vi "PICRv1.1.vi"() -> ()   [LabVIEW 2013]
uses:
  <vilib>/userdefined/High Color/IMAQdx.ctl
  <vilib>/LabVIEW Interface for Arduino/Type Defs/Board Type.ctl
  <vilib>/LabVIEW Interface for Arduino/Type Defs/Connection Type.ctl
  <vilib>/vision/driver/NI_Vision_Acquisition_Software.lvlib
  <vilib>/LabVIEW Interface for Arduino/LabVIEW Interface for Arduino.lvlib
panel:
  in  "Enum":enum16{"", "Forward", "Back"}(ring)
  in  "VISA resource":refnum<visa-resource-name>
  in  "Play 2":bool
  in  "Back 2":bool
  in  "Forward 2":bool
  in  "Play":bool
  in  "Back":bool
  in  "Forward":bool
  in  "Speed Control - Brush":dbl(knob) scale=0.0..100.0
  out "Speed - Brush":dbl(knob) scale=0.0..100.0
  in  "Speed Control - Motors":dbl(knob) scale=0.0..100.0
  out "Speed - Motors":dbl(knob) scale=0.0..100.0
  in  "Stop":bool
  out "Image":T1(plugin-control)
  in  "Session In":T2
  # "Motion"
  # "IMU"
  # "Camera"
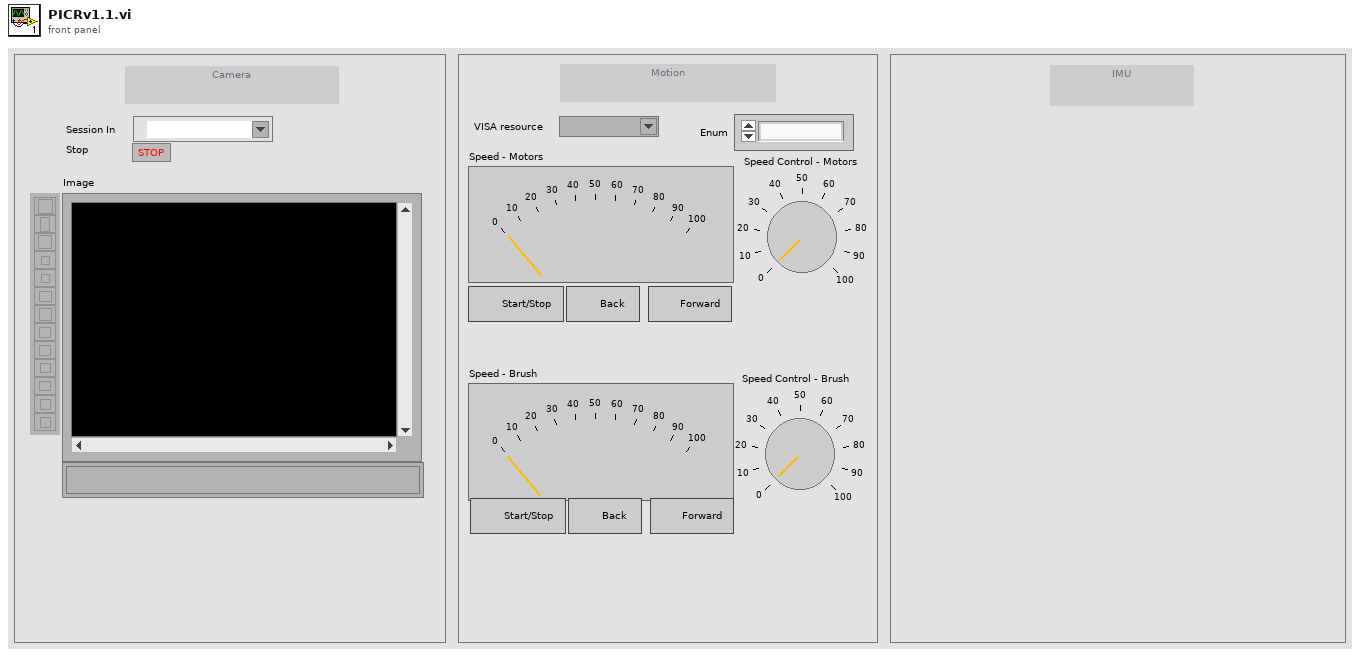
[diagram p1: front panel]
types:
  T1 = typedef "IMAQ Image.ctl" = refnum<image>
  T2 = typedef "IMAQdx.ctl" = refnum<k21>
  T3 = typedef "LabVIEW Interface for Arduino.lvlib/Connection Type.ctl" = enum8{"USB / Serial", "XBEE", "BlueSmirf (Bluetooth)"}
  T4 = typedef "LabVIEW Interface for Arduino.lvlib/Board Type.ctl" = enum16{"Uno", "Dimuelanove w/Atmega 328", "Mega 2560"}
  T5 = typedef "Image Type" = u32
  T6 = typedef "LabVIEW Interface for Arduino.lvlib/Arduino Resource.ctl" = cluster{"VISA resource":refnum<visa-resource-name>, "Board Type":T4, "Connection Type":enum8{"USB / Serial"}, "Bytes Per Packet (15)":u8}
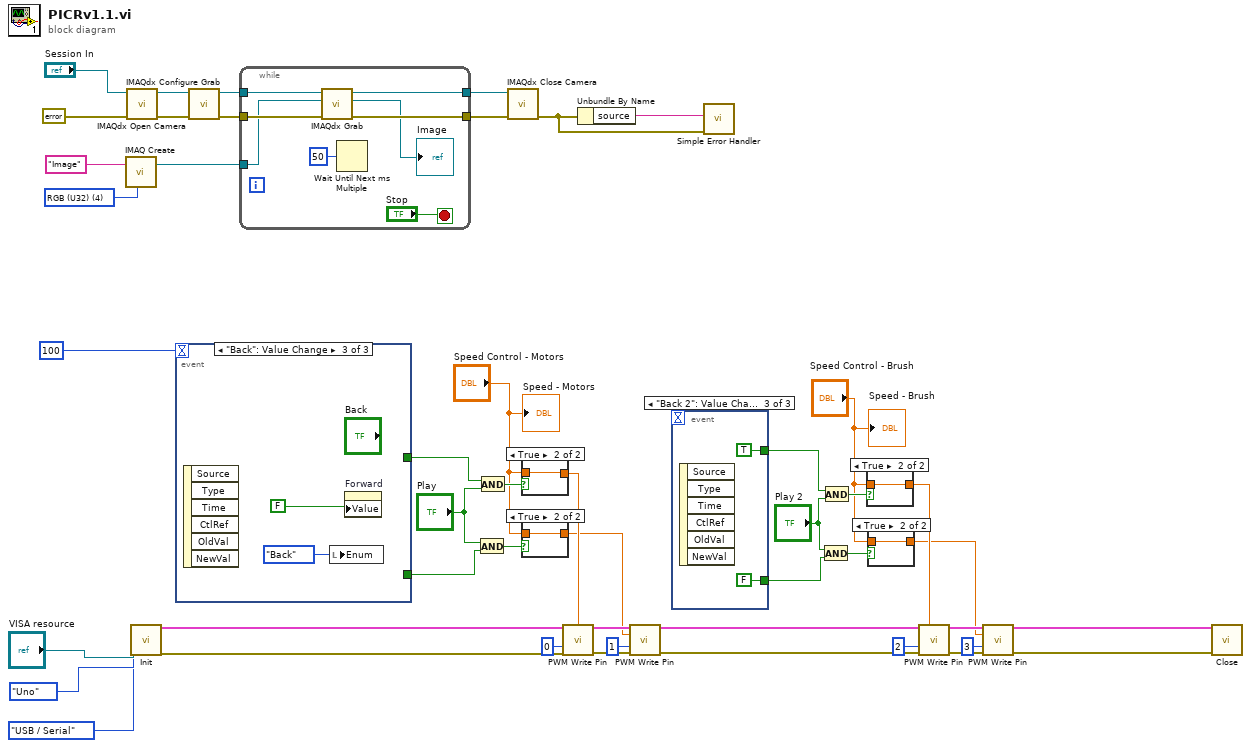
[diagram p0: block diagram]
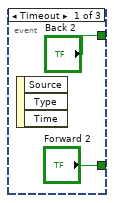
[diagram p2: hidden frame]
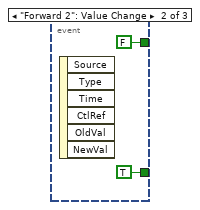
[diagram p3: hidden frame]
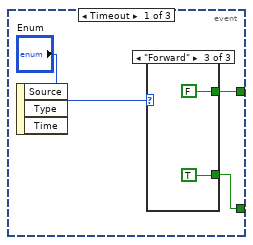
[diagram p4: hidden frame]
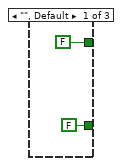
[diagram p5: hidden frame]
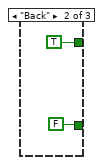
[diagram p6: hidden frame]
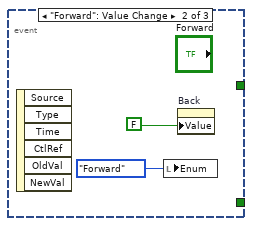
[diagram p7: hidden frame]
diagram:
  w38 = T5 4 items=["Grayscale (U8)", "Grayscale (I16)", "Grayscale (SGL)", "Complex (CSG)", "RGB (U32)", "HSL (U32)", "RGB (U64)", "Grayscale (U16)"] ("Image Type")
  n1 = call "IMAQ Create"("Image Name"="Image", "Image Type"=w38) -> ("New Image"=w37:T1)  [unwired: 3 in, 1 out]
  n2 = call <vilib>:"IMAQdx Open Camera.vi"("error in"=errorcluster {"status"=FALSE, "code"=0, "source"=""}, "Session In"="Session In") -> ("error out"=w42:errorcluster, "Session Out"=w47:T2)  [unwired: 8 in]
  n3 = call <vilib>:"Init.vi"("VISA resource"="VISA resource", "Board Type (Uno)"=Board_Type."Uno", "Connection Type (USB/Serial)"=Connection_Type."USB / Serial") -> ("Arduino Resource"=w25:T6, "error out"=w20:errorcluster)  [unwired: 15 in]
  n4 = event shown="[2] \"Back\": Value Change" {
    selector: _ -> [_ _ _]
    dyn-events: _ -> [_ _ _]
    timeout: 100 -> [_ _ _]
    tunnel: [w49 _ _] -> w34
    tunnel: [w48 _ _] -> w32
    event Timeout {
      n5 = event-data() -> ()  [unwired: 1 in, 3 out]
      n6 = case shown="\"Forward\"" "Enum" {
        tunnel: [FALSE TRUE FALSE] -> w49
        tunnel: [FALSE FALSE TRUE] -> w48
        frame "", Default {
        }
        frame "Back" {
        }
        frame "Forward" {
        }
      }
    }
    event "Forward": Value Change {
      n7 = event-data() -> ()  [unwired: 1 in, 6 out]
      n8 = local write "Enum"(enum16{"", "Forward", "Back"}."Forward") -> ()
      n9 = property on="Back" class="Bool"("Value"=FALSE) -> ()  [unwired: 2 in, 2 out]
    }
    event "Back": Value Change {
      n10 = event-data() -> ()  [unwired: 1 in, 6 out]
      n11 = local write "Enum"(enum16{"", "Forward", "Back"}."Back") -> ()
      n12 = property on="Forward" class="Bool"("Value"=FALSE) -> ()  [unwired: 2 in, 2 out]
    }
  }
  n13 = call <vilib>:"IMAQdx Configure Grab.vi"("error in"=w42, "Session In"=w47) -> ("error out"=w41:errorcluster, "Session Out"=w46:T2)  [unwired: 8 in]
  n14 = while {
    tunnel: w46 -> [w68]
    tunnel: [w67] -> w45
    tunnel: w41 -> [w66]
    tunnel: [w65] -> w40
    tunnel: w37 -> [w64]
    stop <- "Stop" stop-if-true
    n15 = call <vilib>:"IMAQdx Grab.vi"("error in"=w66, "Image In"=w64, "Session In"=w68) -> ("error out"=w65:errorcluster, "Image Out"=→"Image":T1, "Session Out"=w67:T2)  [unwired: 5 in, 1 out]
    n16 = Wait Until Next ms Multiple(millisecond multiple=u32 50) -> ()  [unwired: 1 out]
  }
  n17 = And(x="Play", y=w32) -> (x .and. y?=w9:bool)
  n18 = And(x=w34, y="Play") -> (x .and. y?=w11:bool)
  n19 = call <vilib>:"IMAQdx Close Camera.vi"("error in"=w40, "Session In"=w45) -> ("error out"=w35:errorcluster)  [unwired: 9 in]
  n20 = case shown="True" w11 {
    tunnel: [_ w69] -> w10
    tunnel: "Speed Control - Motors" -> [_ w69]
    frame False {
    }
    frame True {
    }
  }
  n21 = case shown="True" w9 {
    tunnel: "Speed Control - Motors" -> [_ w70]
    tunnel: [_ w70] -> w7
    frame False {
    }
    frame True {
    }
  }
  n22 = call <vilib>:"PWM Write Pin.vi"("Arduino Resource"=w25, "Duty Cycle (0 - 255)"=w10, "PWM Pin (3)"=u8 0, "error in"=w20) -> ("Arduino Resource"=w24:T6, "error out"=w19:errorcluster)  [unwired: 10 in]
  n23 = Unbundle By Name(w35) -> ("source"=w36:string)
  n24 = call <vilib>:"PWM Write Pin.vi"("Arduino Resource"=w24, "Duty Cycle (0 - 255)"=w7, "PWM Pin (3)"=u8 1, "error in"=w19) -> ("Arduino Resource"=w23:T6, "error out"=w18:errorcluster)  [unwired: 10 in]
  n25 = event shown="[2] \"Back 2\": Value Change" {
    selector: _ -> [_ _ _]
    dyn-events: _ -> [_ _ _]
    timeout: _ -> [_ _ _]
    tunnel: ["Forward 2" TRUE ("Forward 2") FALSE ("Forward 2")] -> w31
    tunnel: ["Back 2" FALSE ("Back 2") TRUE ("Back 2")] -> w29
    event Timeout {
      n26 = event-data() -> ()  [unwired: 1 in, 3 out]
    }
    event "Forward 2": Value Change {
      n27 = event-data() -> ()  [unwired: 1 in, 6 out]
    }
    event "Back 2": Value Change {
      n28 = event-data() -> ()  [unwired: 1 in, 6 out]
    }
  }
  n29 = call <vilib>:"Simple Error Handler.vi"("error source (\" \")"=w36, "error in (no error)"=w35) -> ()  [unwired: 3 in, 5 out]
  n30 = And(x="Play 2", y=w31) -> (x .and. y?=w6:bool)
  n31 = And(x=w29, y="Play 2") -> (x .and. y?=w5:bool)
  n32 = case shown="True" w5 {
    tunnel: "Speed Control - Brush" -> [_ w77]
    tunnel: [_ w77] -> w4
    frame False {
    }
    frame True {
    }
  }
  n33 = case shown="True" w6 {
    tunnel: "Speed Control - Brush" -> [_ w78]
    tunnel: [_ w78] -> w2
    frame False {
    }
    frame True {
    }
  }
  n34 = call <vilib>:"PWM Write Pin.vi"("Arduino Resource"=w23, "Duty Cycle (0 - 255)"=w4, "PWM Pin (3)"=u8 2, "error in"=w18) -> ("Arduino Resource"=w22:T6, "error out"=w17:errorcluster)  [unwired: 10 in]
  n35 = call <vilib>:"PWM Write Pin.vi"("Arduino Resource"=w22, "Duty Cycle (0 - 255)"=w2, "PWM Pin (3)"=u8 3, "error in"=w17) -> ("Arduino Resource"=w21:T6, "error out"=w16:errorcluster)  [unwired: 10 in]
  n36 = call <vilib>:"Close.vi"("Arduino Resource"=w21, "error in"=w16) -> ()  [unwired: 13 in, 1 out]
  "Speed - Motors" <- "Speed Control - Motors"
  "Speed - Brush" <- "Speed Control - Brush"
